vi "Lockin Noise Measurement.vi"(8 "error in (no error)":errorcluster, 9 "Iterations":i32, 10 "time constant (s)":dbl format="%#_6p") -> (0 "error out":errorcluster, 2 "Noise = Volts[amps]/Sqrt(Hz)":dbl[](array[numeric]) format="%#_6p")   [LabVIEW 2019]
uses:
  src/Instrument.Lockin/Typedefs/Results Type--Enum.ctl
  src/Instrument.Lockin/Instrument.Lockin.lvclass
  <vilib>/ptbypt/NI_PtbyPt.lvlib
panel:
  out "3. <|X - <X>|>":T1(graph)
  out "2. X - <X>":T1(graph)
  in  "stop":bool
  out "1. <X>":T1(graph)
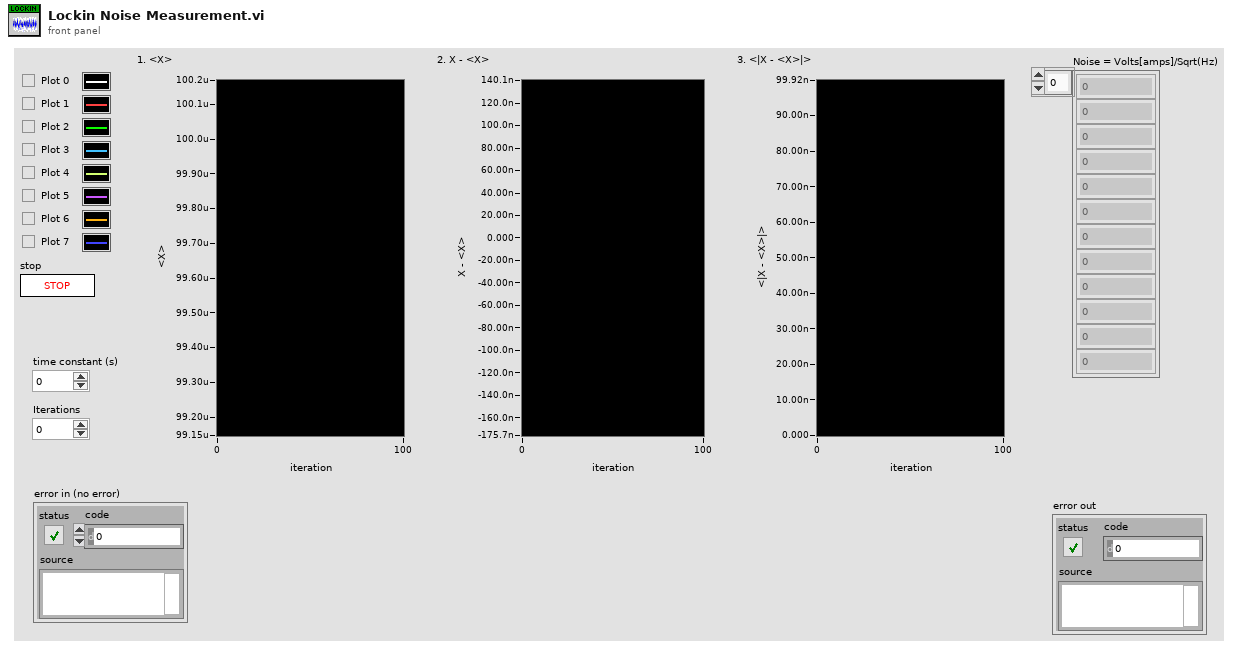
[diagram p1: front panel]
types:
  T1 = cluster{"[0]":dbl, "[1]":dbl, "[2]":dbl, "[3]":dbl, "[4]":dbl, "[5]":dbl, "[6]":dbl, "[7]":dbl, "[8]":dbl}
  T2 = cluster{"[0]":dbl, "[1]":dbl, "[2]":dbl, "[3]":dbl, "[4]":dbl, "[5]":dbl, "[6]":dbl, "[7]":dbl, "[8]":dbl}[]
  T3 = typedef "Instrument.Lockin.lvlib/Instrument.Lockin.lvclass/Results Type--Enum.ctl" = enum16{"X", "Y", "R", "Theta", "Mean"}
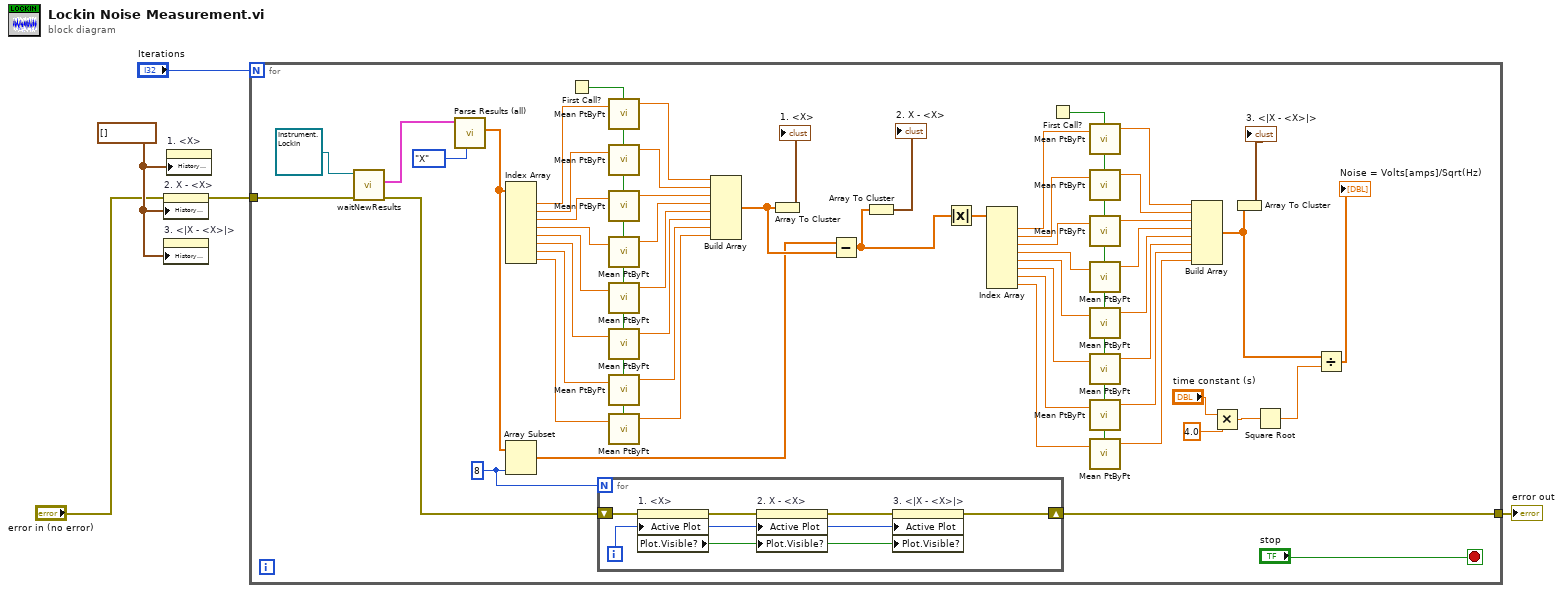
[diagram p0: block diagram]
diagram:
  w4 = T2 [] ("History Data")
  n1 = property on="2. X - <X>" class="WFChart (strict)"(error in="error in (no error)", "History Data"=w4) -> (error out=w5:errorcluster)  [unwired: 1 in, 1 out]
  n2 = property on="3. <|X - <X>|>" class="WFChart (strict)"("History Data"=w4) -> ()  [unwired: 2 in, 2 out]
  n3 = property on="1. <X>" class="WFChart (strict)"("History Data"=w4) -> ()  [unwired: 2 in, 2 out]
  n4 = for {
    N: "Iterations" -> [_]
    tunnel: w5 -> [w11]
    tunnel: [w14] -> w2
    stop <- "stop" stop-if-true
    w10 = 8 ("length")
    n5 = call-dynamic "waitNewResults.vi"("error in (no error)"=w11, "Instrument.Lockin in"=refnum<class "Instrument.Lockin.lvclass"> refnum) -> ("error out"=w12:errorcluster, "Results (Dictionary)"=w9:cluster{"key":string, "value":dbl}[])  [unwired: 7 in, 1 out]
    n6 = call "Parse Results (all).vi"("Type"=Results_Type--Enum."X", "Results (Dictionary)"=w9) -> ("Data"=w7:dbl[])  [unwired: 6 in, 3 out]
    n7 = Index Array(array=w7) -> (element #1=w61:dbl, element #2=w60:dbl, element #3=w59:dbl, element #4=w58:dbl, element #5=w57:dbl, element #6=w56:dbl, element #7=w55:dbl, element #8=w54:dbl)  [unwired: 8 in]
    n8 = Array Subset(array=w7, length=w10) -> (w41:dbl[])  [unwired: 1 in]
    n9 = First Call?() -> (First Call?: T/F=w42:bool)
    n10 = for {
      N: w10 -> [_]
      shift-right: [w62] -> w14
      shift-left: w12 -> [w67]
      i -> [w64]
      n11 = property on="1. <X>" class="WFChart (strict)"(error in=w67, "Active Plot"=w64) -> (error out=w66:errorcluster, "Plot.Visible?"=w65:bool)  [unwired: 1 in, 1 out]
      n12 = property on="2. X - <X>" class="WFChart (strict)"(error in=w66, "Active Plot"=w64, "Plot.Visible?"=w65) -> (error out=w63:errorcluster)  [unwired: 1 in, 1 out]
      n13 = property on="3. <|X - <X>|>" class="WFChart (strict)"(error in=w63, "Active Plot"=w64, "Plot.Visible?"=w65) -> (error out=w62:errorcluster)  [unwired: 1 in, 1 out]
    }
    n14 = call <vilib>:"Mean PtByPt.vi"("x"=w61, "initialize"=w42) -> ("mean"=w53:dbl)  [unwired: 2 in, 1 out]
    n15 = call <vilib>:"Mean PtByPt.vi"("x"=w60, "initialize"=w42) -> ("mean"=w52:dbl)  [unwired: 2 in, 1 out]
    n16 = call <vilib>:"Mean PtByPt.vi"("x"=w59, "initialize"=w42) -> ("mean"=w51:dbl)  [unwired: 2 in, 1 out]
    n17 = call <vilib>:"Mean PtByPt.vi"("x"=w58, "initialize"=w42) -> ("mean"=w50:dbl)  [unwired: 2 in, 1 out]
    n18 = call <vilib>:"Mean PtByPt.vi"("x"=w57, "initialize"=w42) -> ("mean"=w49:dbl)  [unwired: 2 in, 1 out]
    n19 = call <vilib>:"Mean PtByPt.vi"("x"=w56, "initialize"=w42) -> ("mean"=w48:dbl)  [unwired: 2 in, 1 out]
    n20 = call <vilib>:"Mean PtByPt.vi"("x"=w55, "initialize"=w42) -> ("mean"=w47:dbl)  [unwired: 2 in, 1 out]
    n21 = call <vilib>:"Mean PtByPt.vi"("x"=w54, "initialize"=w42) -> ("mean"=w46:dbl)  [unwired: 2 in, 1 out]
    n22 = Build Array(w53, w52, w51, w50, w49, w48, w47, w46) -> (w44:dbl[])
    n23 = Array To Cluster(array=w44) -> (cluster=→"1. <X>":T1)
    n24 = Subtract(x=w41, y=w44) -> (x-y=w21:dbl[])
    n25 = Array To Cluster(array=w21) -> (cluster=→"2. X - <X>":T1)
    n26 = Absolute Value(x=w21) -> (abs(x)=w22:dbl[])
    n27 = Index Array(array=w22) -> (element #1=w24:dbl, element #2=w25:dbl, element #3=w26:dbl, element #4=w27:dbl, element #5=w28:dbl, element #6=w29:dbl, element #7=w30:dbl, element #8=w31:dbl)  [unwired: 8 in]
    n28 = First Call?() -> (First Call?: T/F=w40:bool)
    n29 = call <vilib>:"Mean PtByPt.vi"("x"=w24, "initialize"=w40) -> ("mean"=w32:dbl)  [unwired: 2 in, 1 out]
    n30 = call <vilib>:"Mean PtByPt.vi"("x"=w25, "initialize"=w40) -> ("mean"=w33:dbl)  [unwired: 2 in, 1 out]
    n31 = call <vilib>:"Mean PtByPt.vi"("x"=w26, "initialize"=w40) -> ("mean"=w34:dbl)  [unwired: 2 in, 1 out]
    n32 = call <vilib>:"Mean PtByPt.vi"("x"=w27, "initialize"=w40) -> ("mean"=w35:dbl)  [unwired: 2 in, 1 out]
    n33 = call <vilib>:"Mean PtByPt.vi"("x"=w28, "initialize"=w40) -> ("mean"=w36:dbl)  [unwired: 2 in, 1 out]
    n34 = call <vilib>:"Mean PtByPt.vi"("x"=w29, "initialize"=w40) -> ("mean"=w37:dbl)  [unwired: 2 in, 1 out]
    n35 = call <vilib>:"Mean PtByPt.vi"("x"=w30, "initialize"=w40) -> ("mean"=w38:dbl)  [unwired: 2 in, 1 out]
    n36 = call <vilib>:"Mean PtByPt.vi"("x"=w31, "initialize"=w40) -> ("mean"=w39:dbl)  [unwired: 2 in, 1 out]
    n37 = Build Array(w32, w33, w34, w35, w36, w37, w38, w39) -> (w20:dbl[])
    n38 = Multiply(x="time constant (s)", y=4.0) -> (x*y=w17:dbl)
    n39 = Array To Cluster(array=w20) -> (cluster=→"3. <|X - <X>|>":T1)
    n40 = Square Root(x=w17) -> (sqrt(x)=w16:dbl)
    n41 = Divide(x=w20, y=w16) -> (x/y=→"Noise = Volts[amps]/Sqrt(Hz)":dbl[])
  }
  "error out" <- w2
